vi "Read FieldCurrentRatio (T_A).vi"(8 "error in (no error)":errorcluster, 11 "PS Driver in":refnum<class "PS Driver.lvclass">) -> (0 "error out":errorcluster, 2 "FieldCurrentRatio (T/A)":dbl, 3 "PS Driver out":refnum<class "PS Driver.lvclass">)   [LabVIEW 2024, in "PS Driver.lvlib" / "PS Driver.lvclass"]
uses:
  PS Driver.lvclass
  PS Driver.lvclass/PS Driver.ctl
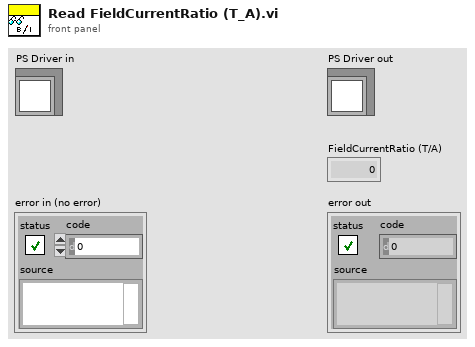
[diagram p1: front panel]
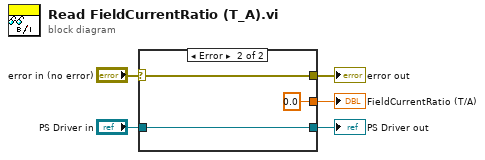
[diagram p0: block diagram]
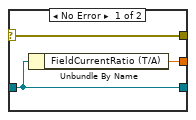
[diagram p2: hidden frame]
diagram:
  n1 = case shown="Error" "error in (no error)" {
    selector: "error in (no error)" -> [w8 w10]
    tunnel: [w8 w10] -> w4
    tunnel: [w7 w11] -> w2
    tunnel: "PS Driver in" -> [w7 w11]
    tunnel: [w6 0.0 ("FieldCurrentRatio (T/A)")] -> w1
    frame No Error {
      n2 = Unbundle By Name(w7) -> ("FieldCurrentRatio (T/A)"=w6:dbl)
    }
    frame Error {
    }
  }
  "error out" <- w4
  "PS Driver out" <- w2
  "FieldCurrentRatio (T/A)" <- w1
